vi "express vi曲线.vi"() -> ()   [LabVIEW 2018]
uses:
  <vilib>/express/express arith-compare/Formula/XNode/ExpressFormulaBlockNode.xnode
panel:
  in  "停止":bool
  out "XY Graph":cluster{"X":dbl[], "Y":dbl[]}[](graph) caption="XY图"
  in  "X":i32(slide) scale=0.0..10.0
  in  "Y":dbl(slide) scale=0.0..10.0
  in  "trim":i32(slide) scale=0.0..10.0
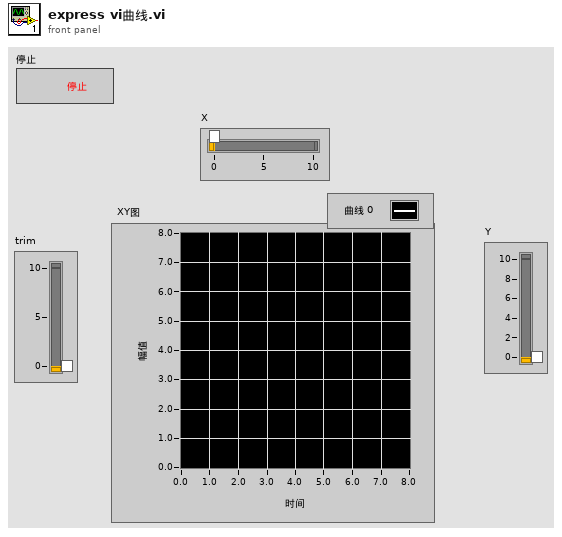
[diagram p1: front panel]
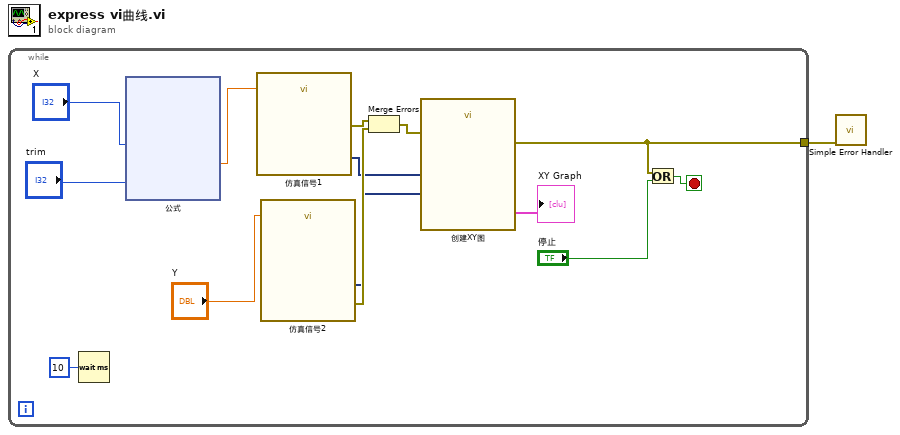
[diagram p0: block diagram]
diagram:
  n1 = while {
    tunnel: [w3] -> w1
    stop <- w4 stop-if-true
    n2 = Wait (ms)(milliseconds to wait=u32 10 ("等待时间（毫秒）")) -> ()  [unwired: 1 out]
    n3 = xnode "公式"("X"="X", "Trim"="trim") -> ("结果"=w8:dbl)  [unwired: 1 in, 1 out]
    n4 = call "仿真信号1"("Frequency"=w8) -> ("正弦"=w6:dynamicdata, "error out"=w12:errorcluster)  [unwired: 13 in]
    n5 = call "仿真信号2"("Frequency"="Y") -> ("正弦"=w5:dynamicdata, "error out"=w7:errorcluster)  [unwired: 13 in]
    n6 = Merge Errors(w12, w7) -> (w10:errorcluster)
    n7 = call "创建XY图"("error in (no error)"=w10, "Y Input"=w5, "X Input"=w6) -> ("error out"=w3:errorcluster, "XY Graph"=→"XY Graph":cluster{"X":dbl[], "Y":dbl[]}[])  [unwired: 7 in]
    n8 = Or(x=w3, y="停止") -> (x .or. y?=w4:bool)
  }
  n9 = call <vilib>:"Simple Error Handler.vi"("error in (no error)"=w1) -> ()  [unwired: 4 in, 5 out]
